vi "LS330_WRITE.vi"(8 "error in":errorcluster, 10 "Input Cluster":T2, 11 "VISA resource name":refnum<visa-resource-name>) -> (0 "error out":errorcluster, 3 "VISA resource name out":refnum<visa-resource-name>)   [LabVIEW 2021]
uses:
  LS330_Setting_Cluster.ctl
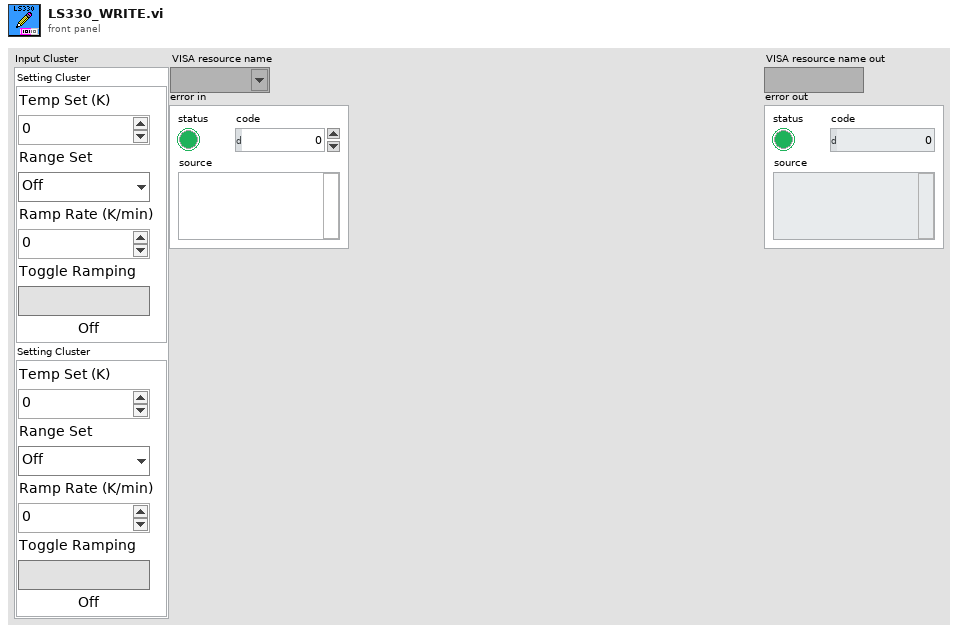
[diagram p1: front panel]
types:
  T1 = typedef "LS330_Setting_Cluster.ctl" = cluster{"Set Temp":dbl, "Set Range":enum16{"Off", "Low", "Medium", "High"}, "Set Ramp Rate":dbl, "Toggle Ramping":bool}
  T2 = cluster{"Setting Cluster":T1, "Setting Cluster":T1}
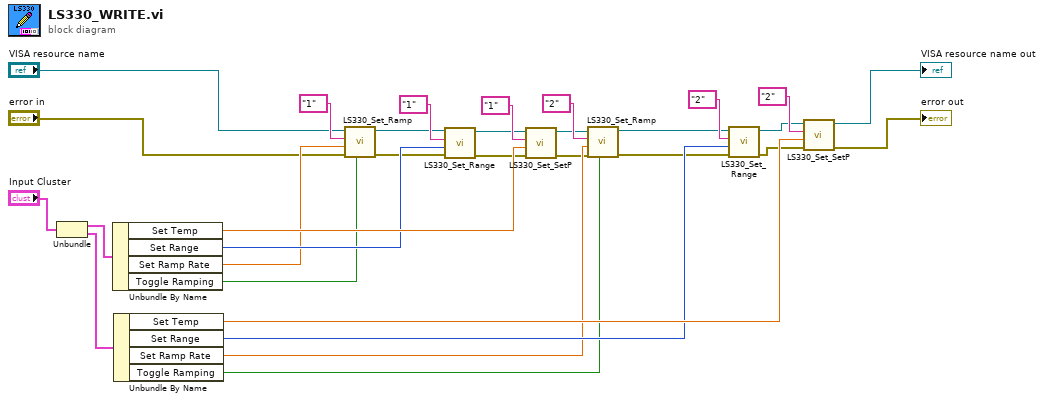
[diagram p0: block diagram]
diagram:
  n1 = Unbundle("Input Cluster") -> ("Setting Cluster"=w30:T1, "Setting Cluster"=w22:T1)
  n2 = Unbundle By Name(w30) -> ("Set Temp"=w28:dbl, "Set Range"=w26:enum16{"Off", "Low", "Medium", "High"}, "Set Ramp Rate"=w24:dbl, "Toggle Ramping"=w23:bool)
  n3 = Unbundle By Name(w22) -> ("Set Temp"=w18:dbl, "Set Range"=w17:enum16{"Off", "Low", "Medium", "High"}, "Set Ramp Rate"=w16:dbl, "Toggle Ramping"=w15:bool)
  n4 = call "LS330_Set_Ramp.vi"("Ramp Toggle"=w23, "error in"="error in", "Ramp Rate"=w24, "Heater"="1", "VISA resource name"="VISA resource name") -> ("error out"=w11:errorcluster, "VISA resource name out"=w12:refnum<visa-resource-name>)  [unwired: 4 in]
  n5 = call "LS330_Set_Range.vi"("error in"=w11, "Range"=w26, "Heater"="1", "VISA resource name"=w12) -> ("error out"=w9:errorcluster, "VISA resource name out"=w10:refnum<visa-resource-name>)  [unwired: 5 in]
  n6 = call "LS330_Set_SetP.vi"("error in"=w9, "Set Temp (K)"=w28, "Heater"="1", "VISA resource name"=w10) -> ("error out"=w7:errorcluster, "VISA resource name out"=w8:refnum<visa-resource-name>)  [unwired: 5 in]
  n7 = call "LS330_Set_Ramp.vi"("Ramp Toggle"=w15, "error in"=w7, "Ramp Rate"=w16, "Heater"="2", "VISA resource name"=w8) -> ("error out"=w5:errorcluster, "VISA resource name out"=w6:refnum<visa-resource-name>)  [unwired: 4 in]
  n8 = call "LS330_Set_Range.vi"("error in"=w5, "Range"=w17, "Heater"="2", "VISA resource name"=w6) -> ("error out"=w3:errorcluster, "VISA resource name out"=w4:refnum<visa-resource-name>)  [unwired: 5 in]
  n9 = call "LS330_Set_SetP.vi"("error in"=w3, "Set Temp (K)"=w18, "Heater"="2", "VISA resource name"=w4) -> ("error out"=→"error out":errorcluster, "VISA resource name out"=→"VISA resource name out":refnum<visa-resource-name>)  [unwired: 5 in]
